vi "OutputList2Info.vi"(0 "Output List String":string, 1 "Format":enum16{"ASCII", "Binary"}(ring)=enum."Binary") -> (2 "Output Bytes":i32[](array[numeric]), 3 "Output Titles":string[](array[string]), 4 "#Reads Out":i32, 5 "Ends with Terminator?":bool)   [LabVIEW 2012]
doc: "Takes direct output from the Polhemus Fastrak. Interprets the output list returned after the 'O#\\r' command, where # is the station number. Returns the number of bytes and name of each output segment during normal operation. This allows for precise reading and interpretation of output later.\n\n'Format' refers to the current fastrak setting, either 'ASCII' or 'Binary', set by the the 'F' and 'f' commands to the Fastrak respectively. Default is Binary."
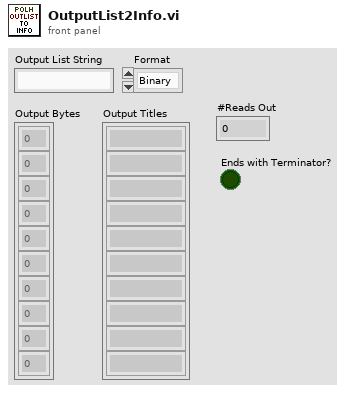
[diagram p1: front panel]
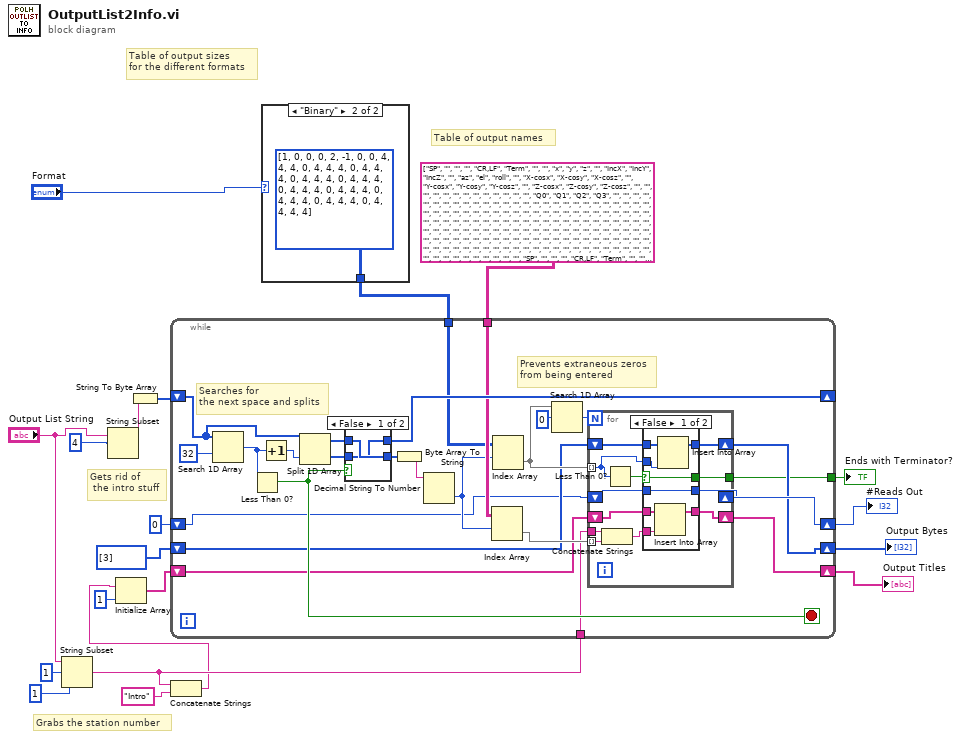
[diagram p0: block diagram]
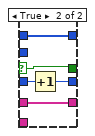
[diagram p2: hidden frame]
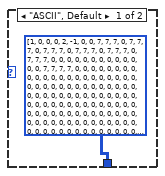
[diagram p4: hidden frame]
diagram:
  # "Grabs the station number"
  # "Gets rid of\n the intro stuff"
  # "Table of output names"
  # "Table of output sizes\nfor the different formats"
  n1 = String Subset(string="Output List String", offset (0)=1, length (rest)=1 ("length (rest)")) -> (substring=w5:string)
  n2 = String Subset(string="Output List String", offset (0)=4) -> (substring=w19:string)  [unwired: 1 in]
  n3 = String To Byte Array(string=w19) -> (unsigned byte array=w18:u8[])
  n4 = Concatenate Strings(w5, "Intro") -> (w4:string)
  n5 = Initialize Array(w4, 1 ("dimension size")) -> (w3:string[])
  n6 = case shown="\"Binary\"" "Format" {
    tunnel: [i32[][] [[1, 0, 0, 0], [2, -1, 0, 0], [7, 7, 7, 0], [7, 7, 7, 0], [7, 7, 7, 0], [7, 7, 7, 0], [7, 7, 7, 0], [7, 7, 7, 0], [0, 0, 0, 0], [0, 0, 0, 0], [0, 0, 0, 0], [7, 7, 7, 7], [0, 0, 0, 0], [0, 0, 0, 0], [0, 0, 0, 0], [0, 0, 0, 0], [0, 0, 0, 0], [0, 0, 0, 0], [0, 0, 0, 0], [0, 0, 0, 0], [0, 0, 0, 0], [0, 0, 0, 0], [0, 0, 0, 0], [0, 0, 0, 0], [0, 0, 0, 0], [0, 0, 0, 0], [0, 0, 0, 0], [0, 0, 0, 0], [0, 0, 0, 0], [0, 0, 0, 0], [0, 0, 0, 0], [0, 0, 0, 0], [0, 0, 0, 0], [0, 0, 0, 0], [0, 0, 0, 0], [0, 0, 0, 0], [0, 0, 0, 0], [0, 0, 0, 0], [0, 0, 0, 0], [0, 0, 0, 0], [0, 0, 0, 0], [0, 0, 0, 0], [0, 0, 0, 0], [0, 0, 0, 0], [0, 0, 0, 0], [0, 0, 0, 0], [0, 0, 0, 0], [0, 0, 0, 0], [0, 0, 0, 0], [0, 0, 0, 0], [1, 0, 0, 0], [2, -1, 0, 0], [13, 13, 13, 0], [13, 13, 13, 0], [13, 13, 13, 0], [13, 13, 13, 0], [13, 13, 13, 0], [13, 13, 13, 0], [0, 0, 0, 0], [0, 0, 0, 0], [0, 0, 0, 0], [13, 13, 13, 13]] i32[][] [[1, 0, 0, 0], [2, -1, 0, 0], [4, 4, 4, 0], [4, 4, 4, 0], [4, 4, 4, 0], [4, 4, 4, 0], [4, 4, 4, 0], [4, 4, 4, 0], [4, 4, 4, 0], [4, 4, 4, 0], [4, 4, 4, 0], [4, 4, 4, 4]]] -> w16
    frame "ASCII", Default {
    }
    frame "Binary" {
    }
  }
  n7 = while {
    shift-right: [w43] -> _
    shift-left: w18 -> [w46]
    tunnel: string[][] [["SP", "", "", ""], ["CR,LF", "Term", "", ""], ["x", "y", "z", ""], ["IncX", "IncY", "IncZ", ""], ["az", "el", "roll", ""], ["X-cosx", "X-cosy", "X-cosz", ""], ["Y-cosx", "Y-cosy", "Y-cosz", ""], ["Z-cosx", "Z-cosy", "Z-cosz", ""], ["", "", "", ""], ["", "", "", ""], ["", "", "", ""], ["Q0", "Q1", "Q2", "Q3"], ["", "", "", ""], ["", "", "", ""], ["", "", "", ""], ["", "", "", ""], ["", "", "", ""], ["", "", "", ""], ["", "", "", ""], ["", "", "", ""], ["", "", "", ""], ["", "", "", ""], ["", "", "", ""], ["", "", "", ""], ["", "", "", ""], ["", "", "", ""], ["", "", "", ""], ["", "", "", ""], ["", "", "", ""], ["", "", "", ""], ["", "", "", ""], ["", "", "", ""], ["", "", "", ""], ["", "", "", ""], ["", "", "", ""], ["", "", "", ""], ["", "", "", ""], ["", "", "", ""], ["", "", "", ""], ["", "", "", ""], ["", "", "", ""], ["", "", "", ""], ["", "", "", ""], ["", "", "", ""], ["", "", "", ""], ["", "", "", ""], ["", "", "", ""], ["", "", "", ""], ["", "", "", ""], ["", "", "", ""], ["SP", "", "", ""], ["CR,LF", "Term", "", ""], ["x", "y", "z", ""], ["Incx", "Incy", "IncZ", ""], ["az", "el", "roll", ""], ["X-cosx", "X-cosy", "X-cosz", ""], ["Y-cosx", "Y-cosy", "Y-cosz", ""], ["Z-cosx", "Z-cosy", "Z-cosz", ""], ["", "", "", ""], ["", "", "", ""], ["", "", "", ""], ["Q0", "Q1", "Q2", "Q3"]] -> [w39]
    tunnel: w16 -> [w38]
    shift-right: [w25] -> w11
    shift-left: i32[] [3] -> [w30]
    shift-right: [w28] -> w12
    shift-left: w3 -> [w29]
    shift-right: [w26] -> w13
    shift-left: 0 -> [w27]
    tunnel: w5 -> [w24]
    tunnel: [w23] -> w1
    stop <- w45 stop-if-true
    # "Prevents extraneous zeros\nfrom being entered"
    # "Searches for\nthe next space and splits"
    n8 = Search 1D Array(1D array=w46, element=u8 32) -> (index of element=w35:i32)  [unwired: 1 in]
    n9 = Less Than 0?(x=w35) -> (x < 0?=w45:bool)
    n10 = Increment(x=w35) -> (x+1=w34:i32)
    n11 = Split 1D Array(array=w46, index=w34) -> (first subarray=w44:u8[], second subarray=w42:u8[])
    n12 = case shown="False" w45 {
      tunnel: w44 -> [w74 w76]
      tunnel: [w73 w76] -> w43
      tunnel: w42 -> [w73 w75]
      tunnel: [w74 w75] -> w41
      frame False {
      }
      frame True {
      }
    }
    n13 = Byte Array To String(unsigned byte array=w41) -> (string=w40:string)
    n14 = Decimal String To Number(string=w40) -> (number=w37:i32)  [unwired: 2 in, 1 out]
    n15 = Index Array(array=w39, index (row)=w37) -> (element=w36:string[])  [unwired: 1 in]
    n16 = Index Array(array=w38, index (row)=w37) -> (element=w33:i32[])  [unwired: 1 in]
    n17 = Search 1D Array(1D array=w33, element=0) -> (index of element=w31:i32)  [unwired: 1 in]
    n18 = for {
      N: w31 -> [_]
      tunnel: w33 -> [w51] mode=indexing
      tunnel: w36 -> [w55] mode=indexing
      shift-right: [w50] -> w25
      shift-left: w30 -> [w52]
      shift-right: [w49] -> w28
      shift-left: w29 -> [w54]
      shift-right: [w57] -> w26
      shift-left: w27 -> [w58]
      tunnel: w24 -> [w56]
      tunnel: [w48] -> w23
      n19 = Concatenate Strings(w56, w55) -> (w53:string)
      n20 = Less Than 0?(x=w51) -> (x < 0?=w59:bool)
      n21 = case shown="False" w59 {
        selector: w59 -> [w60 w68]
        tunnel: w58 -> [w67 w72]
        tunnel: [w67 w71] -> w57
        tunnel: w54 -> [w66 w70]
        tunnel: w53 -> [w65 _]
        tunnel: w52 -> [w64 w69]
        tunnel: w51 -> [w63 _]
        tunnel: [w62 w69] -> w50
        tunnel: [w61 w70] -> w49
        tunnel: [w60 w68] -> w48
        frame False {
          n22 = Insert Into Array(array=w66, new element=w65) -> (w61:string[])  [unwired: 1 in]
          n23 = Insert Into Array(array=w64, new element=w63) -> (w62:i32[])  [unwired: 1 in]
        }
        frame True {
          n24 = Increment(x=w72) -> (x+1=w71:i32)
        }
      }
    }
  }
  "#Reads Out" <- w13
  "Output Titles" <- w12
  "Output Bytes" <- w11
  "Ends with Terminator?" <- w1
